vi "Microscopy.TriggerOptions.vi"(7 "Trigger In":bool, 8 "Data Valid in":bool=TRUE, 9 "Trigger Falling Edge Detect":bool, 10 "Trigger Type":T1, 11 "Software Trigger from Host":bool) -> (0 "Data Valid out":bool, 3 "trigger edge":bool)   [LabVIEW 2014]
uses:
  Adapter Module Specific/Trigger Type.ctl
panel:
  # "Copyright 2014 Vidrio Technologies\nScanImage 5 software is licensed under the Apache License, Version 2.0 (the \"License\"); you may not use any files contained\nwithin the ScanImage 5 release except in compliance with the License. You may obtain a copy of the License at\n http://www.apache.org/licenses/LICENSE-2.0\nUnless required by applicable law or agreed to in writing, software distributed under the License is distributed on an\n\"AS IS\" BASIS, WITHOUT WARRANTIES OR CONDITIONS OF ANY KIND, either express or implied. See the License for the\n specific language governing permissions and limitations under the License."
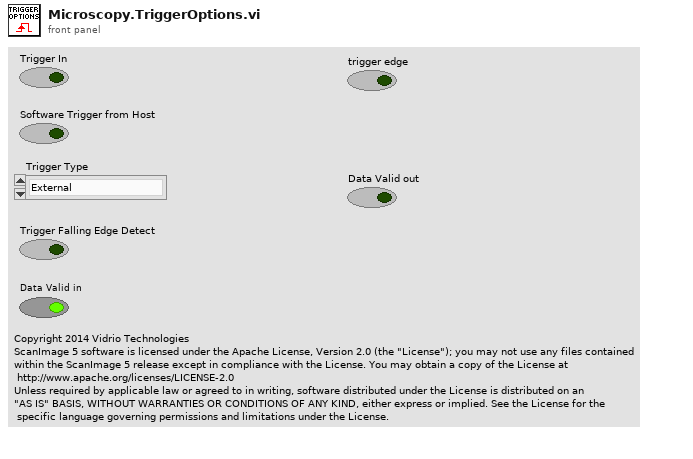
[diagram p1: front panel]
types:
  T1 = typedef "Trigger Type.ctl" = enum8{"External", "Software", "Immediate", "External or Software", "None"}
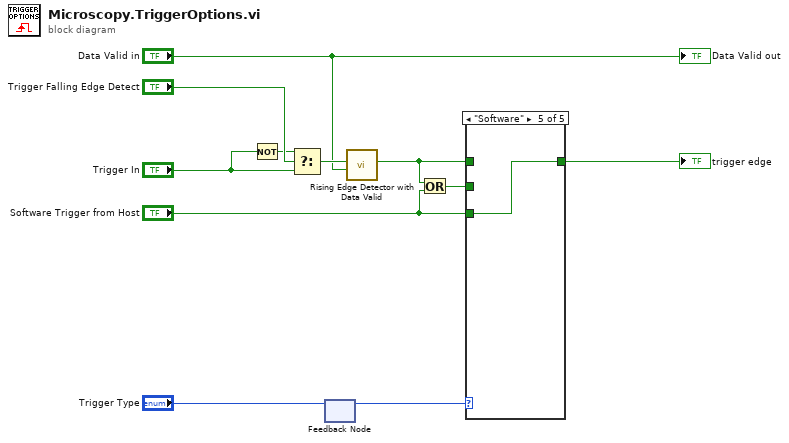
[diagram p0: block diagram]
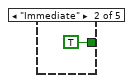
[diagram p3: hidden frame]
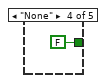
[diagram p5: hidden frame]
diagram:
  n1 = Not(x="Trigger In") -> (.not. x?=w6:bool)
  n2 = Select(t=w6, s="Trigger Falling Edge Detect", f="Trigger In") -> (s? t:f=w7:bool)
  n3 = feedback #1() -> (w5:T1)  [unwired: 1 in]
  n4 = feedback-in #1("Trigger Type") -> ()
  n5 = call "Rising Edge Detector with Data Valid.vi"("Data Valid"="Data Valid in", "signal"=w7) -> ("edge detected"=w3:bool)  [unwired: 9 in]
  n6 = Or(x=w3, y="Software Trigger from Host") -> (x .or. y?=w1:bool)
  n7 = case shown="\"Software\"" w5 {
    tunnel: "Software Trigger from Host" -> [_ _ _ _ w16]
    tunnel: [w12 TRUE ("edge detected") w14 FALSE ("Software Trigger from Host") w16] -> w11
    tunnel: w3 -> [w12 _ _ _ _]
    tunnel: w1 -> [_ _ w14 _ _]
    frame "External", Default {
    }
    frame "Immediate" {
    }
    frame "External or Software" {
    }
    frame "None" {
    }
    frame "Software" {
    }
  }
  "trigger edge" <- w11
  "Data Valid out" <- "Data Valid in"
